vi "Run Test (Object Array).vi"(4 "timeout (2000 ms)":i32=2000, 5 "Test Report":refnum<class "Test Report.lvclass">, 6 "Verbose":bool, 7 "Report Path":path, 8 "error in":errorcluster, 10 "Objects":refnum<class>[](array[class]), 11 "Interactive (T)":bool=TRUE) -> (0 "error out":errorcluster, 3 "Test Results":refnum<class "Test Result.lvclass">)   [LabVIEW 2013, in "Caraya.lvlib"]
doc: "\"Run Tests\" from an array of class instances:\n- Dynamically discovers Caraya unit tests in multiple classes and runs them\n- Outputs results in a UI ans/or Test Report (J-Unit or text)\n\n(Not compatible with RT targets or RunTime Engine)"
uses:
  Caraya.lvlib
  classes/Test Report/Test Report.lvclass
  classes/Test Result/Test Result.lvclass
  classes/Test Runner.Class/Test Runner.Class.lvclass
  classes/Test Runner/Test Runner.lvclass
  classes/Test Runner.Collection/Test Runner.Collection.lvclass
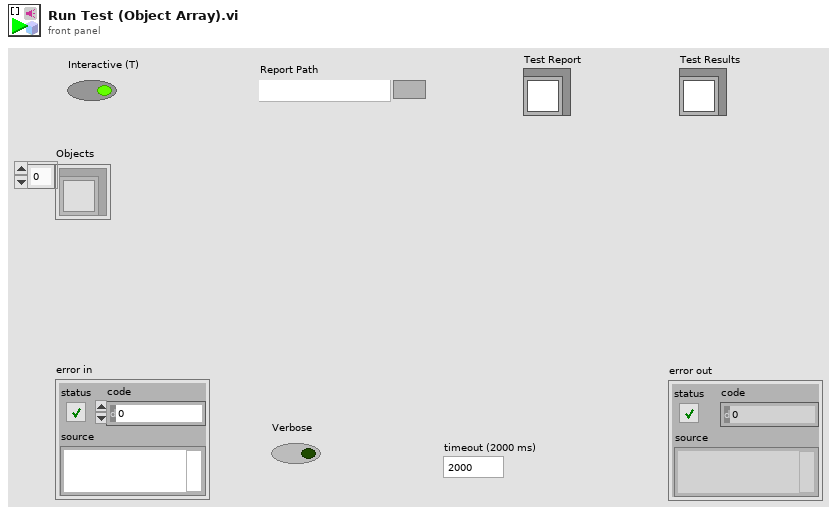
[diagram p1: front panel]
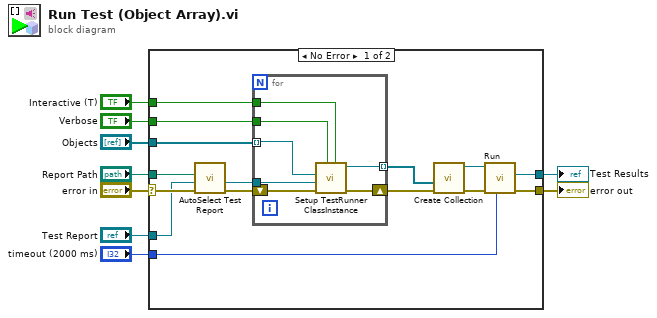
[diagram p0: block diagram]
diagram:
  n1 = case shown="No Error" "error in" {
    selector: "error in" -> [w21 w32]
    tunnel: [w24 w32] -> w9
    tunnel: "Verbose" -> [w23 _]
    tunnel: "Interactive (T)" -> [w22 _]
    tunnel: "Test Report" -> [w19 _]
    tunnel: "Objects" -> [w18 _]
    tunnel: "Report Path" -> [w20 _]
    tunnel: "timeout (2000 ms)" -> [w11 _]
    tunnel: [w10 _] -> w1
    frame No Error {
      n2 = call "AutoSelect Test Report.vi"("error in (no error)"=w21, "Test Report in"=w19, "Report Path"=w20) -> ("error out"=w17:errorcluster, "Test Report out"=w12:refnum<class "Test Report.lvclass">)  [unwired: 7 in]
      n3 = for {
        tunnel: w23 -> [w31]
        tunnel: w22 -> [w30]
        tunnel: w18 -> [w27] mode=indexing
        tunnel: [w26] -> w16 mode=indexing
        shift-right: [w25] -> w15
        shift-left: w17 -> [w28]
        tunnel: w12 -> [w29]
        n4 = call "Setup TestRunner ClassInstance.vi"("Interactive (T)"=w30, "Verbose (F)"=w31, "error in (no error)"=w28, "Test Report"=w29, "Instance"=w27) -> ("error out"=w25:errorcluster, "Test Runner.Class out"=w26:refnum<class "Test Runner.Class.lvclass">)  [unwired: 5 in]
      }
      n5 = call "Create Collection.vi"("error in (no error)"=w15, "Test Runners"=w16) -> ("error out"=w14:errorcluster, "Test Runner.Collection out"=w13:refnum<class "Test Runner.Collection.lvclass">)  [unwired: 8 in]
      n6 = call "Run.vi"("timeout"=w11, "error in (no error)"=w14, "Test Runner in"=w13) -> ("error out"=w24:errorcluster, "Test Suite Results"=w10:refnum<class "Test Result.lvclass">)  [unwired: 6 in, 1 out]
    }
    frame Error {
    }
  }
  "error out" <- w9
  "Test Results" <- w1
